vi "Init.vi"(9 "Event":refnum<class "Event.lvclass">, 10 "Self Event Alias":string) -> (3 "Create Event Msg Strategy out":refnum<class "Create Event Msg Strategy.lvclass">)   [LabVIEW 2021, in "jettl Msg Create Event.lvlib" / "Create Event Msg Strategy.lvclass"]
uses:
  Create Event Msg Strategy.lvclass
  jettl/Event/Event.lvclass
  Create Event Msg Strategy.lvclass/Create Event Msg Strategy.ctl
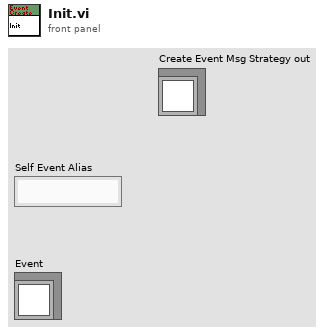
[diagram p1: front panel]
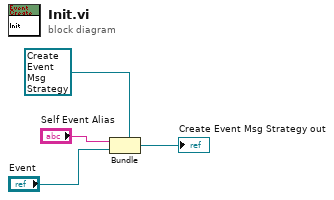
[diagram p0: block diagram]
diagram:
  n1 = Bundle(cluster=refnum<class "Create Event Msg Strategy.lvclass"> refnum ("Event Create Msg out"), "Self Event Alias", "Event") -> (→"Create Event Msg Strategy out":refnum<class "Create Event Msg Strategy.lvclass">)
